vi "intSubstract.vi"(8 "Error in (no error)":errorcluster, 10 "Int2 in":refnum<class "IntClass.lvclass">, 11 "Int1 in":refnum<class "IntClass.lvclass">) -> (0 "Error out":errorcluster, 1 "Timing":u32, 3 "Int1 - Int2":refnum<class "IntClass.lvclass">)   [LabVIEW 2011, in "IntClass.lvclass"]
uses:
  IntClass.lvclass
  IntClass.lvclass/IntClass.ctl
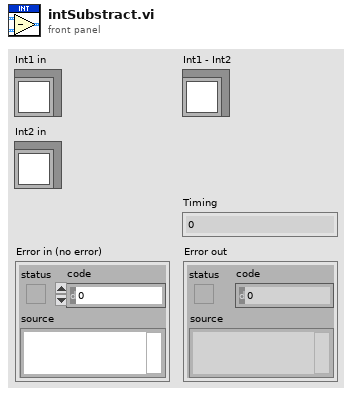
[diagram p1: front panel]
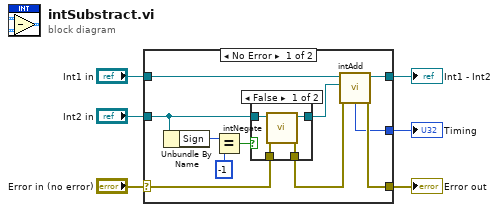
[diagram p0: block diagram]
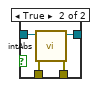
[diagram p2: hidden frame]
diagram:
  n1 = case shown="No Error" "Error in (no error)" {
    selector: "Error in (no error)" -> [w13 w26]
    tunnel: [w9 w26] -> w5
    tunnel: "Int1 in" -> [w12 _]
    tunnel: "Int2 in" -> [w15 _]
    tunnel: [w8 _] -> w2
    tunnel: [w7 _] -> w1
    frame No Error {
      n2 = Unbundle By Name(w15) -> ("Sign"=w17:i8)
      n3 = Equal?(x=w17, y=i8 -1) -> (x = y?=w14:bool)
      n4 = case shown="False" w14 {
        tunnel: w15 -> [w20 w25]
        tunnel: w13 -> [w19 w24]
        tunnel: [w18 w23] -> w10
        tunnel: [w21 w22] -> w11
        frame False {
          n5 = call "intNegate.vi"("Error in (no error)"=w19, "Int in"=w20) -> ("Error out"=w18:errorcluster, "Int out"=w21:refnum<class "IntClass.lvclass">)  [unwired: 8 in]
        }
        frame True {
          n6 = call "intAbs.vi"("Error in (no error)"=w24, "Int in"=w25) -> ("Error out"=w23:errorcluster, "Int out"=w22:refnum<class "IntClass.lvclass">)  [unwired: 8 in]
        }
      }
      n7 = call "intAdd.vi"("Error in (no error)"=w10, "Int2 in"=w11, "Int1 in"=w12) -> ("Error out"=w9:errorcluster, "Timing"=w7:u32, "Int1 + Int2"=w8:refnum<class "IntClass.lvclass">)  [unwired: 6 in]
    }
    frame Error {
    }
  }
  "Int1 - Int2" <- w2
  "Error out" <- w5
  "Timing" <- w1
